vi "Execute.vi"(8 "error in":errorcluster, 11 "Display Data in":refnum<class "Display Data.lvclass">) -> (0 "error out":errorcluster, 1 "Next Step?":bool, 2 "MSG":string, 3 "Display Data out":refnum<class "Display Data.lvclass">)   [LabVIEW 2013, in "Display Data.lvclass"]
uses:
  Display Data.lvclass
  Display.vi
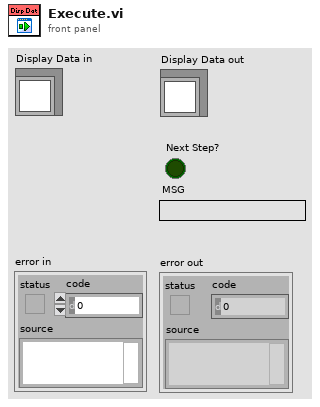
[diagram p1: front panel]
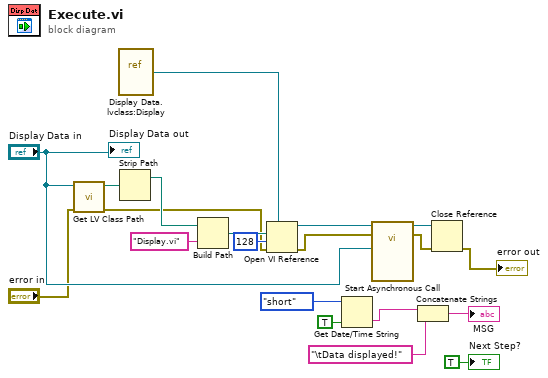
[diagram p0: block diagram]
diagram:
  n1 = call <vilib>:"Get LV Class Path.vi"("error in (no error)"="error in", "object"="Display Data in") -> ("error out"=w2:errorcluster, "class path"=w19:path)  [unwired: 8 in]
  n2 = vi-ref "Display Data.lvclass:Display.vi"() -> (w16:refnum<vi>)
  n3 = Strip Path(path=w19) -> (stripped path=w18:path)  [unwired: 1 out]
  n4 = Build Path(base path=w18, name or relative path="Display.vi") -> (appended path=w15:path)
  n5 = Open VI Reference(type specifier VI Refnum (for type only)=w16, vi path=w15, options=128, error in (no error)=w2) -> (vi reference=w13:refnum<vi>, error out=w12:errorcluster)  [unwired: 2 in]
  n6 = Get Date/Time String(date format (0)=enum16{"short", "long", "abbreviated"}."short", want seconds? (F)=TRUE) -> (time string=w6:string)  [unwired: 1 in, 1 out]
  n7 = call-by-ref "Start Asynchronous Call"(reference=w13, error in=w12, "Display Data"="Display Data in") -> (reference out=w10:refnum<vi>, error out=w9:errorcluster)  [unwired: 11 in]
  n8 = Concatenate Strings(w6, "\tData displayed!" ("MSG")) -> (→"MSG":string)
  n9 = Close Reference(reference=w10, error in (no error)=w9) -> (error out=→"error out":errorcluster)
  "Display Data out" <- "Display Data in"
  "Next Step?" <- TRUE ("Next Step?")
